vi "RESTful Header Mode To Text.vi"(1 "Header Mode":bool) -> (0 "Boolean Text":string)   [LabVIEW 2020]
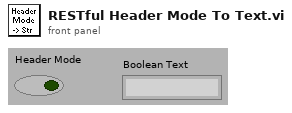
[diagram p1: front panel]
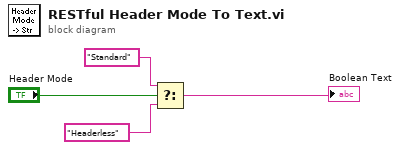
[diagram p0: block diagram]
diagram:
  n1 = Select(t="Standard", s="Header Mode", f="Headerless") -> (s? t:f=→"Boolean Text":string)
